vi "SetButtonValue.vi"(8 "error in (no error)":errorcluster, 9 "value (true)":bool=TRUE, 10 "label":string, 11 "Buttons":refnum<vi>[](array[refnum])) -> (0 "error out":errorcluster, 3 "Buttons out":refnum<vi>[](array[refnum]))   [LabVIEW 2018, in "CarWashTestCases.lvclass"]
uses:
  CarWashTestCases.lvclass
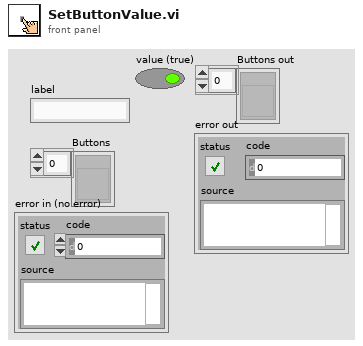
[diagram p1: front panel]
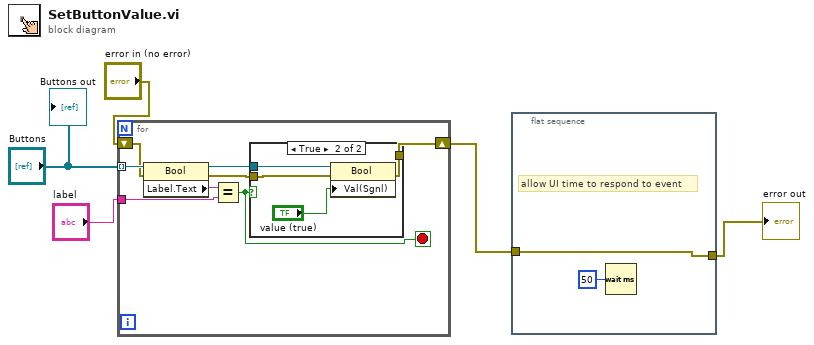
[diagram p0: block diagram]
diagram:
  n1 = for {
    tunnel: "Buttons" -> [w10] mode=indexing
    tunnel: "label" -> [w12]
    shift-right: [w7] -> w2
    shift-left: "error in (no error)" -> [w9]
    stop <- w6 stop-if-true
    n2 = property class="Bool"(reference=w10, error in=w9) -> (reference out=w11:refnum<vi>, error out=w8:errorcluster, "Label.Text"=w13:string)
    n3 = Equal?(x=w13, y=w12) -> (x = y?=w6:bool)
    n4 = case shown="True" w6 {
      tunnel: w11 -> [_ w18]
      tunnel: w8 -> [w14 w17]
      tunnel: [w14 w16] -> w7
      frame False {
      }
      frame True {
        n5 = property class="Bool"(reference=w18, error in=w17, "Val(Sgnl)"="value (true)") -> (error out=w16:errorcluster)  [unwired: 1 out]
      }
    }
  }
  n6 = flat-sequence {
    tunnel: w2 -> [w19]
    tunnel: [w19] -> w1
    frame #0 {
      # "allow UI time to respond to event"
      n7 = Wait (ms)(milliseconds to wait=u32 50) -> ()  [unwired: 1 out]
    }
  }
  "Buttons out" <- "Buttons"
  "error out" <- w1
